vi "getpropiertiesainput.vi"() -> (1 "Array 3":u32[](array[numeric]), 2 "Array 2":u32[](array[numeric]), 3 "Array":u32[](array[numeric]))   [LabVIEW 2013]
uses:
  <vilib>/rvi/eio/common/nirviEmuTemplatePropertyGet_noerrors.vi
  <vilib>/eio/EIOPropertyNode/EIOPropertyNode.xnode
  <vilib>/rvi/eio/common/nirviEmuTemplatePropertyGet_errors.vi
  <vilib>/rvi/eio/common/nirviEmuTemplatePropertySet_errors.vi
  <vilib>/rvi/eio/common/nirviEmuTemplatePropertySet_noerrors.vi
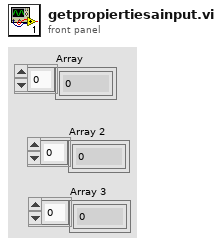
[diagram p1: front panel]
types:
  T1 = cluster{"LSB Weight (+/- 10V range)":i32, "Offset (+/- 10V range)":i32}
  T2 = cluster{"Linearization Coefficient 0":u32, "Linearization Coefficient 1":u32, "Linearization Coefficient 2":u32, "Linearization Coefficient 3":u32}
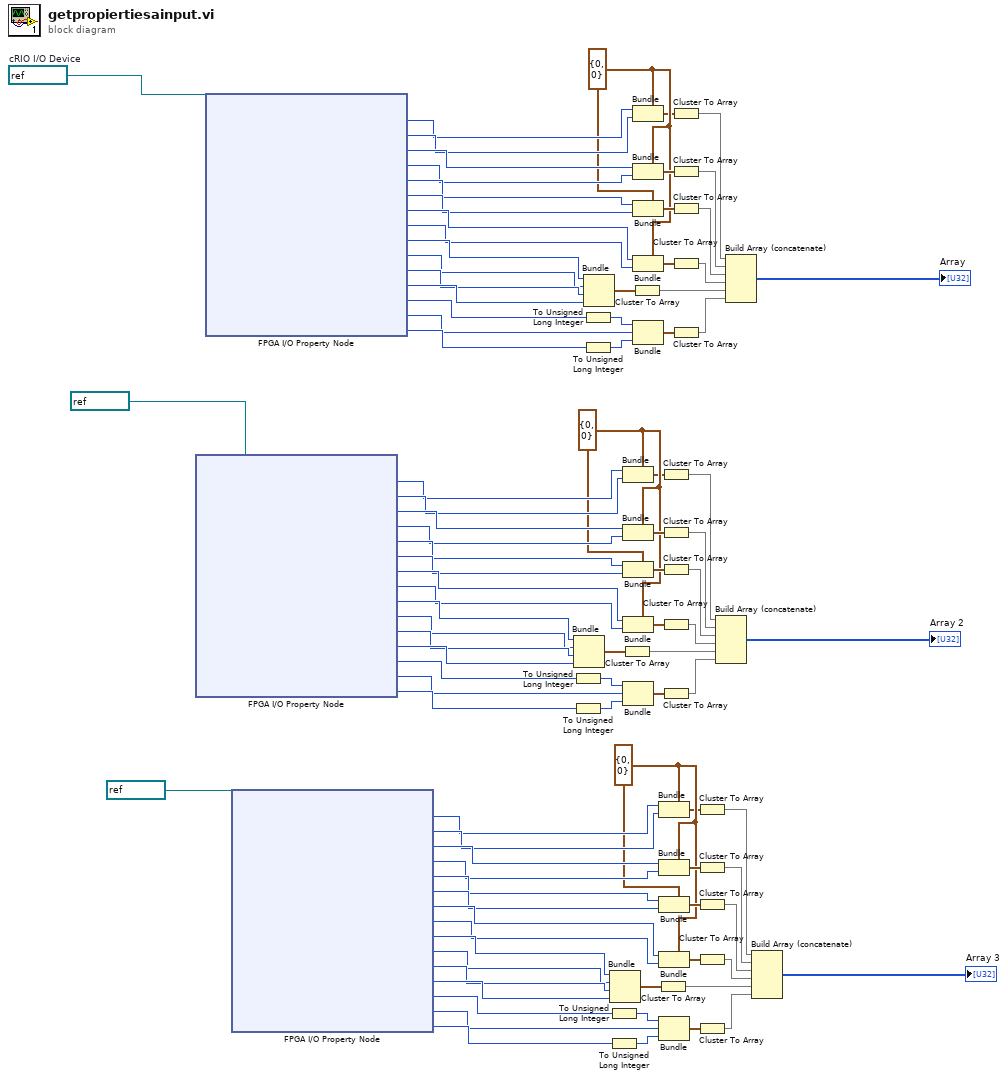
[diagram p0: block diagram]
diagram:
  w1 = refnum<k21> "Mod1"  # cRIO I/O Device
  w4 = T1 {"LSB Weight (+/- 10V range)"=0, "Offset (+/- 10V range)"=0} ("cluster")
  w36 = T1 {"LSB Weight (+/- 10V range)"=0, "Offset (+/- 10V range)"=0} ("cluster")
  w68 = T1 {"LSB Weight (+/- 10V range)"=0, "Offset (+/- 10V range)"=0} ("cluster")
  n1 = xnode "FPGA I/O Property Node"("FPGA I/O In"=refnum<k21> "Mod2" ("cRIO I/O Device 2")) -> ("LSB Weight (+/- 10V range)"=w51:u32, "Offset (+/- 10V range)"=w52:i32, "LSB Weight (+/- 5V range)"=w53:u32, "Offset (+/- 5V range)"=w54:i32, "LSB Weight (+/- 1V range)"=w55:u32, "Offset (+/- 1V range)"=w56:i32, "LSB Weight (+/- 200mV range)"=w57:u32, "Offset (+/- 200mV range)"=w58:i32, "Linearization Coefficient 0"=w59:u32, "Linearization Coefficient 1"=w60:u32, "Linearization Coefficient 2"=w61:u32, "Linearization Coefficient 3"=w62:u32, "Module ID"=w63:u16, "Serial Number"=w64:u32, "Vendor ID"=w65:u16)  [unwired: 1 out]
  n2 = xnode "FPGA I/O Property Node"("FPGA I/O In"=w1) -> ("LSB Weight (+/- 10V range)"=w82:u32, "Offset (+/- 10V range)"=w83:i32, "LSB Weight (+/- 5V range)"=w84:u32, "Offset (+/- 5V range)"=w85:i32, "LSB Weight (+/- 1V range)"=w86:u32, "Offset (+/- 1V range)"=w87:i32, "LSB Weight (+/- 200mV range)"=w88:u32, "Offset (+/- 200mV range)"=w89:i32, "Linearization Coefficient 0"=w90:u32, "Linearization Coefficient 1"=w91:u32, "Linearization Coefficient 2"=w92:u32, "Linearization Coefficient 3"=w93:u32, "Module ID"=w94:u16, "Serial Number"=w95:u32, "Vendor ID"=w96:u16)  [unwired: 1 out]
  n3 = xnode "FPGA I/O Property Node"("FPGA I/O In"=refnum<k21> "Mod3" ("cRIO I/O Device 3")) -> ("LSB Weight (+/- 10V range)"=w19:u32, "Offset (+/- 10V range)"=w20:i32, "LSB Weight (+/- 5V range)"=w21:u32, "Offset (+/- 5V range)"=w22:i32, "LSB Weight (+/- 1V range)"=w23:u32, "Offset (+/- 1V range)"=w24:i32, "LSB Weight (+/- 200mV range)"=w25:u32, "Offset (+/- 200mV range)"=w26:i32, "Linearization Coefficient 0"=w27:u32, "Linearization Coefficient 1"=w28:u32, "Linearization Coefficient 2"=w29:u32, "Linearization Coefficient 3"=w30:u32, "Module ID"=w31:u16, "Serial Number"=w32:u32, "Vendor ID"=w33:u16)  [unwired: 1 out]
  n4 = To Unsigned Long Integer(number=w63) -> (unsigned 32bit integer=w45:u32)
  n5 = To Unsigned Long Integer(number=w65) -> (unsigned 32bit integer=w46:u32)
  n6 = Bundle("Linearization Coefficient 0"=w59, "Linearization Coefficient 1"=w60, "Linearization Coefficient 2"=w61, "Linearization Coefficient 3"=w62) -> (w34:T2)  [unwired: 1 out]
  n7 = To Unsigned Long Integer(number=w94) -> (unsigned 32bit integer=w77:u32)
  n8 = To Unsigned Long Integer(number=w96) -> (unsigned 32bit integer=w78:u32)
  n9 = Bundle("Linearization Coefficient 0"=w90, "Linearization Coefficient 1"=w91, "Linearization Coefficient 2"=w92, "Linearization Coefficient 3"=w93) -> (w66:T2)  [unwired: 1 out]
  n10 = To Unsigned Long Integer(number=w31) -> (unsigned 32bit integer=w13:u32)
  n11 = To Unsigned Long Integer(number=w33) -> (unsigned 32bit integer=w14:u32)
  n12 = Bundle("Linearization Coefficient 0"=w27, "Linearization Coefficient 1"=w28, "Linearization Coefficient 2"=w29, "Linearization Coefficient 3"=w30) -> (w2:T2)  [unwired: 1 out]
  n13 = Cluster To Array(cluster=w34) -> (array=w43:u32[])
  n14 = Bundle(cluster=w36, "LSB Weight (+/- 10V range)"=w51, "Offset (+/- 10V range)"=w52) -> (w35:T1)
  n15 = Bundle(cluster=w36, "LSB Weight (+/- 10V range)"=w53, "Offset (+/- 10V range)"=w54) -> (w37:T1)
  n16 = Bundle(cluster=w36, "LSB Weight (+/- 10V range)"=w55, "Offset (+/- 10V range)"=w56) -> (w38:T1)
  n17 = Bundle(cluster=w36, "LSB Weight (+/- 10V range)"=w57, "Offset (+/- 10V range)"=w58) -> (w39:T1)
  n18 = Bundle(w45, "Serial Number"=w64, w46) -> (w47:cluster{u32, "Serial Number":u32, u32})  [unwired: 1 out]
  n19 = Cluster To Array(cluster=w66) -> (array=w75:u32[])
  n20 = Bundle(cluster=w68, "LSB Weight (+/- 10V range)"=w82, "Offset (+/- 10V range)"=w83) -> (w67:T1)
  n21 = Bundle(cluster=w68, "LSB Weight (+/- 10V range)"=w84, "Offset (+/- 10V range)"=w85) -> (w69:T1)
  n22 = Bundle(cluster=w68, "LSB Weight (+/- 10V range)"=w86, "Offset (+/- 10V range)"=w87) -> (w70:T1)
  n23 = Bundle(cluster=w68, "LSB Weight (+/- 10V range)"=w88, "Offset (+/- 10V range)"=w89) -> (w71:T1)
  n24 = Bundle(w77, "Serial Number"=w95, w78) -> (w79:cluster{u32, "Serial Number":u32, u32})  [unwired: 1 out]
  n25 = Cluster To Array(cluster=w2) -> (array=w11:u32[])
  n26 = Bundle(cluster=w4, "LSB Weight (+/- 10V range)"=w19, "Offset (+/- 10V range)"=w20) -> (w3:T1)
  n27 = Bundle(cluster=w4, "LSB Weight (+/- 10V range)"=w21, "Offset (+/- 10V range)"=w22) -> (w5:T1)
  n28 = Bundle(cluster=w4, "LSB Weight (+/- 10V range)"=w23, "Offset (+/- 10V range)"=w24) -> (w6:T1)
  n29 = Bundle(cluster=w4, "LSB Weight (+/- 10V range)"=w25, "Offset (+/- 10V range)"=w26) -> (w7:T1)
  n30 = Bundle(w13, "Serial Number"=w32, w14) -> (w15:cluster{u32, "Serial Number":u32, u32})  [unwired: 1 out]
  n31 = Cluster To Array(cluster=w35) -> (array=w40:i32[])
  n32 = Cluster To Array(cluster=w37) -> (array=w41:i32[])
  n33 = Cluster To Array(cluster=w38) -> (array=w49:i32[])
  n34 = Cluster To Array(cluster=w39) -> (array=w42:i32[])
  n35 = Cluster To Array(cluster=w47) -> (array=w48:u32[])
  n36 = Cluster To Array(cluster=w67) -> (array=w72:i32[])
  n37 = Cluster To Array(cluster=w69) -> (array=w73:i32[])
  n38 = Cluster To Array(cluster=w70) -> (array=w81:i32[])
  n39 = Cluster To Array(cluster=w71) -> (array=w74:i32[])
  n40 = Cluster To Array(cluster=w79) -> (array=w80:u32[])
  n41 = Cluster To Array(cluster=w3) -> (array=w8:i32[])
  n42 = Cluster To Array(cluster=w5) -> (array=w9:i32[])
  n43 = Cluster To Array(cluster=w6) -> (array=w17:i32[])
  n44 = Cluster To Array(cluster=w7) -> (array=w10:i32[])
  n45 = Cluster To Array(cluster=w15) -> (array=w16:u32[])
  n46 = Build Array (concatenate)(w40, w41, w49, w42, w43, w48) -> (→"Array 2":u32[])
  n47 = Build Array (concatenate)(w72, w73, w81, w74, w75, w80) -> (→"Array":u32[])
  n48 = Build Array (concatenate)(w8, w9, w17, w10, w11, w16) -> (→"Array 3":u32[])
